vi "Set CD Item Property Value.vi"(8 "error in (no error)":errorcluster, 10 "CD Item Ref in":T1 format="%.0x", 11 "String Parameter in":refnum<class "String Parameter.lvclass">) -> (0 "error out":errorcluster, 3 "String Parameter out":refnum<class "String Parameter.lvclass">)   [LabVIEW 2019, in "CD Parameter Manager API.lvlib" / "String Parameter.lvclass"]
uses:
  String Parameter.lvclass
  C:/Repositories/UI-Control-Initializer-API/Source/Parameter Class/Parameter.lvclass
  <vilib>/NI VeriStand/Custom Device API/Custom Device Item Ref.ctl
  Parameter Class/Parameter.lvclass/Parameter.ctl
  String Parameter.lvclass/String Parameter.ctl
  Parameter Class/Member Accessors/Read Control label.vi
  Member Accessors/Read Value.vi
  <vilib>/NI VeriStand/Custom Device API/Set Item Property (String).vi
  <vilib>/NI VeriStand/Custom Device API/Custom Device API.lvlib
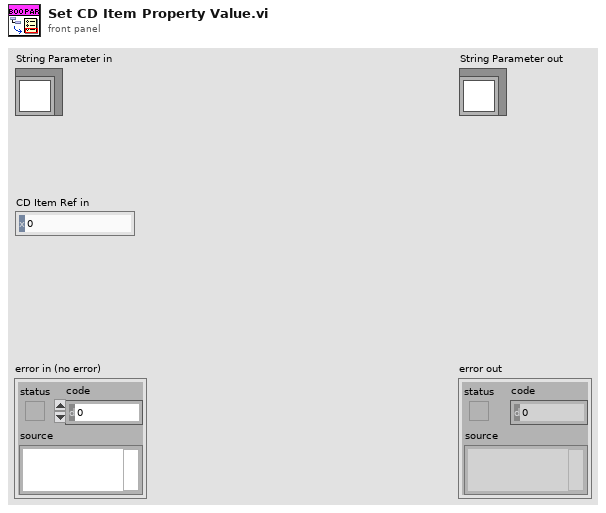
[diagram p1: front panel]
types:
  T1 = typedef "Custom Device API.lvlib/Custom Device Item Ref.ctl" = u64
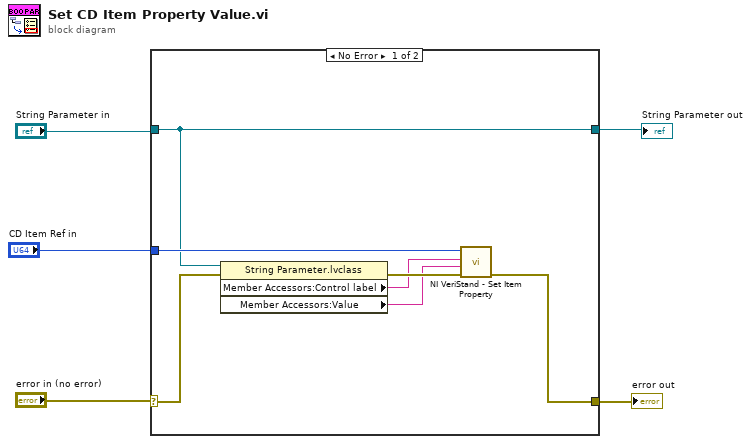
[diagram p0: block diagram]
diagram:
  n1 = case shown="No Error" "error in (no error)" {
    selector: "error in (no error)" -> [w11 w13]
    tunnel: [w6 w13] -> w4
    tunnel: "CD Item Ref in" -> [w12 _]
    tunnel: [w10 w14] -> w5
    tunnel: "String Parameter in" -> [w10 w14]
    frame No Error {
      n2 = property class="String Parameter.lvclass"(reference=w10, error in=w11) -> (error out=w9:errorcluster, "Member Accessors:Control label"=w8:string, "Member Accessors:Value"=w7:string)  [unwired: 1 out]
      n3 = call-poly <vilib>:"NI VeriStand - Set Item Property.vi"("error in (no error)"=w9, "Value"=w7, "Property Name"=w8, "Item Ref in"=w12) -> ("error out"=w6:errorcluster)  [unwired: 5 in, 2 out]
    }
    frame Error {
    }
  }
  "error out" <- w4
  "String Parameter out" <- w5
